vi "sensor_check.vi"() -> ()   [LabVIEW 2019]
uses:
  System.Speech
panel:
  in  "sensor 2":bool
  in  "sensor1":bool
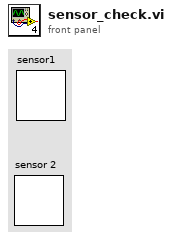
[diagram p1: front panel]
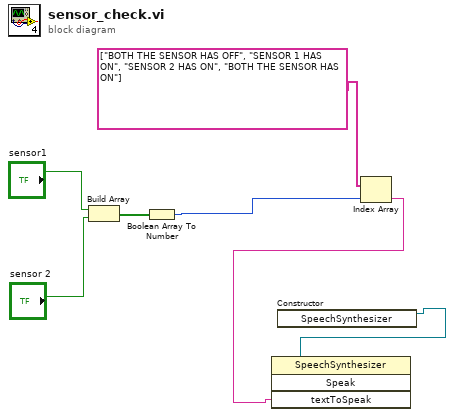
[diagram p0: block diagram]
diagram:
  n1 = Build Array("sensor1", "sensor 2") -> (w4:bool[])
  n2 = Boolean Array To Number(Boolean array=w4) -> (number=w3:u32)
  n3 = constructor class="SpeechSynthesizer"() -> (reference out=w7:refnum<k24>)  [unwired: 3 in, 2 out]
  n4 = Index Array(array=string[] ["BOTH THE SENSOR HAS OFF", "SENSOR 1 HAS ON", "SENSOR 2 HAS ON", "BOTH THE SENSOR HAS ON"], index=w3) -> (element=w1:string)
  n5 = invoke class="SpeechSynthesizer" method="Speak"(reference=w7, "textToSpeak"=w1) -> ()  [unwired: 2 in, 4 out]
